vi "write config ini data.vi"(8 "error in (no error)":errorcluster, 10 "user data in":T2={"sectors"=[], "key names"=[], "values"=[]}, 11 "Refnum in":T1) -> (0 "error out":errorcluster, 3 "Refnum out":T1)   [LabVIEW 2024]
doc: "This VI saves (Write) and retrieves (Read) data from a configuration .ini file, regardless of the number of sectors and the keys in each sector."
uses:
  <vilib>/Utility/config.llb/Config Data RefNum.ctl
  <vilib>/Utility/config.llb/Write Key (String).vi
  <vilib>/Utility/config.llb/NI_LVConfig.lvlib
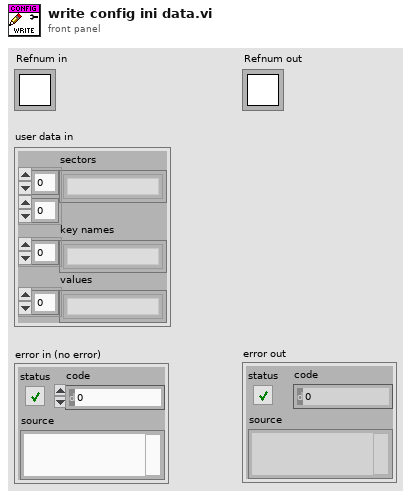
[diagram p1: front panel]
types:
  T1 = typedef "NI_LVConfig.lvlib/Config Data RefNum.ctl" = refnum<k1>
  T2 = cluster{"sectors":string[][], "key names":string[], "values":string[]}
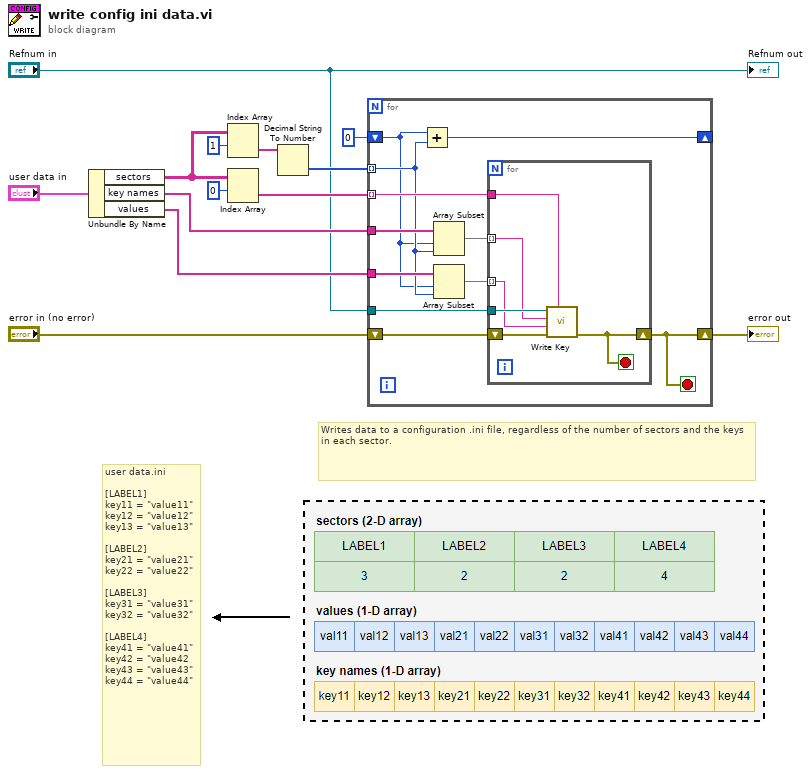
[diagram p0: block diagram]
diagram:
  # "user data.ini\n\n[LABEL1]\nkey11 = \"value11\"\nkey12 = \"value12\"\nkey13 = \"value13\"\n\n[LABEL2]\nkey21 = \"value21\"\nkey22 = \"value22\"\n\n[LABEL3]\nkey31 = \"value31\"\nkey32 = \"value32\"\n\n[LABEL4]\nkey41 = \"value41\"\nkey42 = \"value42\nkey43 = \"value43\"\nkey44 = \"value44\""
  # "Writes data to a configuration .ini file, regardless of the number of sectors and the keys in each sector."
  n1 = Unbundle By Name("user data in") -> ("sectors"=w10:string[][], "key names"=w12:string[], "values"=w11:string[])
  n2 = Index Array(array=w10, index (row)=1) -> (element=w6:string[])  [unwired: 1 in]
  n3 = Index Array(array=w10, index (row)=0) -> (element=w8:string[])  [unwired: 1 in]
  n4 = Decimal String To Number(string=w6) -> (number=w5:i32[])  [unwired: 2 in, 1 out]
  n5 = for {
    tunnel: w11 -> [w17]
    tunnel: w12 -> [w20]
    tunnel: "Refnum in" -> [w23]
    tunnel: w8 -> [w22] mode=indexing
    shift-right: [w21] -> w2
    shift-left: "error in (no error)" -> [w24]
    tunnel: w5 -> [w15] mode=indexing
    shift-right: [w18] -> _
    shift-left: 0 ("sector") -> [w14]
    stop <- w21 stop-if-true
    n6 = Add(x=w14, y=w15) -> (x+y=w18:i32)
    n7 = Array Subset(array=w20, index=w14, length=w15) -> (w19:string[])
    n8 = Array Subset(array=w17, index=w14, length=w15) -> (w16:string[])
    n9 = for {
      tunnel: w23 -> [w30]
      shift-right: [w25] -> w21
      shift-left: w24 -> [w29]
      tunnel: w22 -> [w28]
      tunnel: w19 -> [w27] mode=indexing
      tunnel: w16 -> [w26] mode=indexing
      stop <- w25 stop-if-true
      n10 = call-poly <vilib>:"Write Key.vi"("section"=w28, "error in (no error)"=w29, "value"=w26, "key"=w27, "refnum"=w30) -> ("error out"=w25:errorcluster)  [unwired: 4 in, 2 out]
    }
  }
  "error out" <- w2
  "Refnum out" <- "Refnum in"
